vi "Configure Module.vi"(8 "error in (no error)":errorcluster, 10 "IOV ref in":refnum<k21>, 11 "9213 in":refnum<class "9213.lvclass">) -> (0 "error out":errorcluster, 2 "IOV ref out":refnum<k21>, 3 "9213 out":refnum<class "9213.lvclass">)   [LabVIEW 2019, in "Modules.lvlib" / "9213.lvclass"]
uses:
  9213.lvclass
  9213.lvclass/9213.ctl
  <resource>/objmgr/cRIO.rc
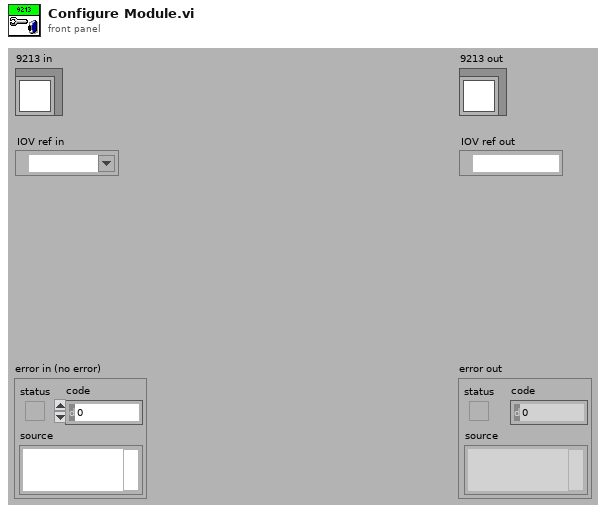
[diagram p1: front panel]
types:
  T1 = typedef "Modules.lvlib/9213.lvclass/Conversion Time.ctl" = u16
  T2 = typedef "Modules.lvlib/9213.lvclass/Measurement Units.ctl" = u8
  T3 = typedef "Modules.lvlib/9213.lvclass/Thermocouple Type.ctl" = u8
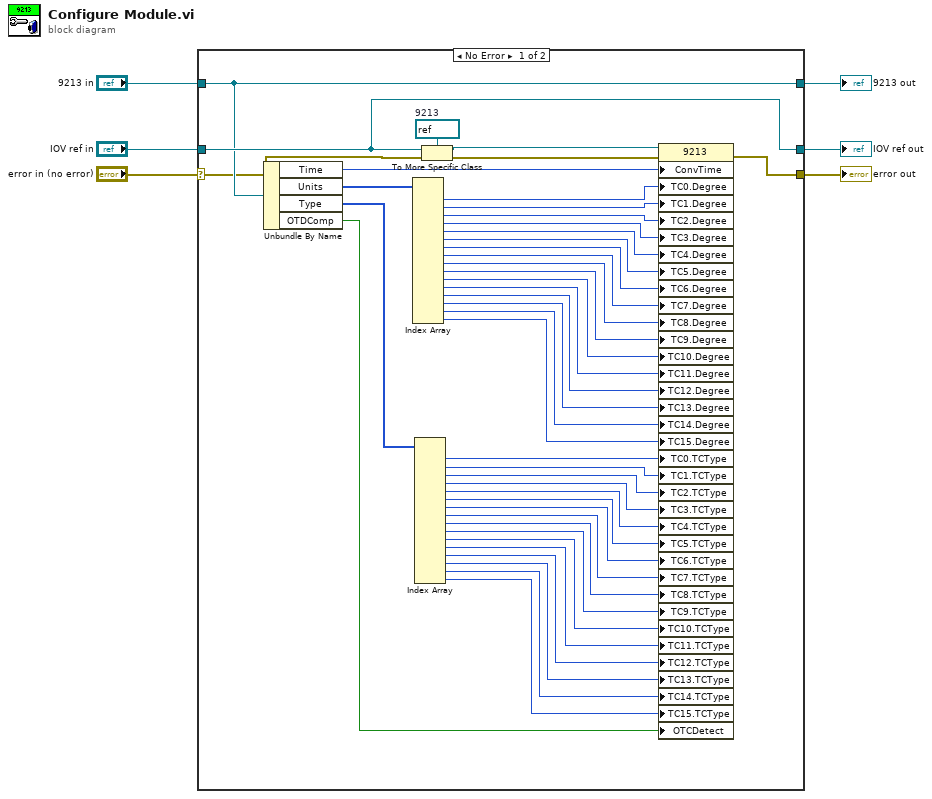
[diagram p0: block diagram]
diagram:
  n1 = case shown="No Error" "error in (no error)" {
    selector: "error in (no error)" -> [w43 w52]
    tunnel: [w47 w52] -> w5
    tunnel: [w44 w51] -> w3
    tunnel: "9213 in" -> [w44 w51]
    tunnel: "IOV ref in" -> [w48 w50]
    tunnel: [w48 w50] -> w1
    frame No Error {
      w42 = refnum<k21> refnum  # 9213
      n2 = Unbundle By Name(w44) -> ("Time"=w49:T1, "Units"=w46:T2[], "Type"=w45:T3[], "OTDComp"=w7:bool)
      n3 = Index Array(array=w46) -> (element #1=w39:T2, element #2=w38:T2, element #3=w37:T2, element #4=w36:T2, element #5=w35:T2, element #6=w34:T2, element #7=w33:T2, element #8=w32:T2, element #9=w31:T2, element #10=w30:T2, element #11=w29:T2, element #12=w28:T2, element #13=w27:T2, element #14=w26:T2, element #15=w25:T2, element #16=w24:T2)  [unwired: 16 in]
      n4 = Index Array(array=w45) -> (element #1=w23:T3, element #2=w22:T3, element #3=w21:T3, element #4=w20:T3, element #5=w19:T3, element #6=w18:T3, element #7=w17:T3, element #8=w16:T3, element #9=w15:T3, element #10=w14:T3, element #11=w13:T3, element #12=w12:T3, element #13=w11:T3, element #14=w10:T3, element #15=w9:T3, element #16=w8:T3)  [unwired: 16 in]
      n5 = To More Specific Class(target class=w42, reference=w48, error in=w43) -> (specific class reference=w41:refnum<k21>, error out=w40:errorcluster)
      n6 = property class="9213"(reference=w41, error in=w40, "ConvTime"=w49, "TC0.Degree"=w39, "TC1.Degree"=w38, "TC2.Degree"=w37, "TC3.Degree"=w36, "TC4.Degree"=w35, "TC5.Degree"=w34, "TC6.Degree"=w33, "TC7.Degree"=w32, "TC8.Degree"=w31, "TC9.Degree"=w30, "TC10.Degree"=w29, "TC11.Degree"=w28, "TC12.Degree"=w27, "TC13.Degree"=w26, "TC14.Degree"=w25, "TC15.Degree"=w24, "TC0.TCType"=w23, "TC1.TCType"=w22, "TC2.TCType"=w21, "TC3.TCType"=w20, "TC4.TCType"=w19, "TC5.TCType"=w18, "TC6.TCType"=w17, "TC7.TCType"=w16, "TC8.TCType"=w15, "TC9.TCType"=w14, "TC10.TCType"=w13, "TC11.TCType"=w12, "TC12.TCType"=w11, "TC13.TCType"=w10, "TC14.TCType"=w9, "TC15.TCType"=w8, "OTCDetect"=w7) -> (error out=w47:errorcluster)  [unwired: 1 out]
    }
    frame Error {
    }
  }
  "error out" <- w5
  "9213 out" <- w3
  "IOV ref out" <- w1
